vi "Microphone_input.vi"() -> ()   [LabVIEW 2013]
uses:
  <vilib>/sound2/lvsound2.llb/Sampling Mode.ctl
  <vilib>/sound2/lvsound2.llb/Sound Input Read (DBL).vi
panel:
  in  "stop":bool
  out "Waveform Graph":waveform(dbl)[](graph)
  in  "number of samples/ch":i32=100000
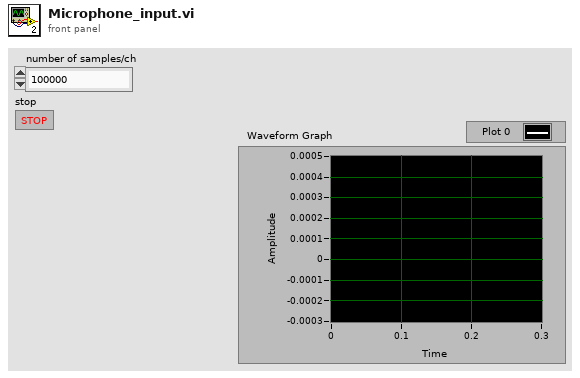
[diagram p1: front panel]
types:
  T1 = typedef "Sampling Mode.ctl" = i32
  T2 = typedef "Sound Input Task ID.ctl" = u32
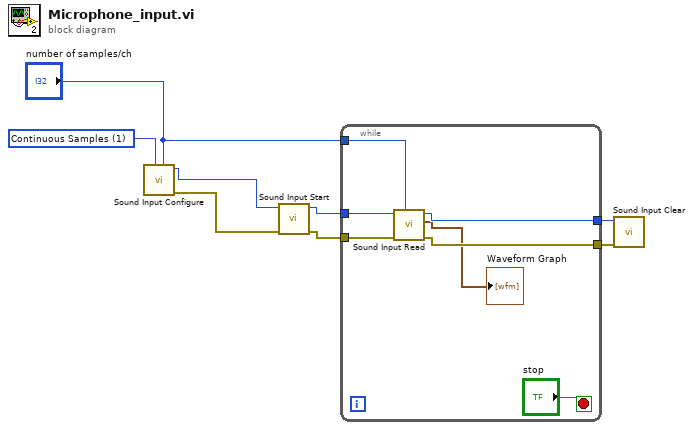
[diagram p0: block diagram]
diagram:
  w2 = T1 1 items=["Finite Samples", "Continuous Samples"] ("sample mode")
  n1 = call <vilib>:"Sound Input Configure.vi"("number of samples/ch"="number of samples/ch", "sample mode"=w2) -> ("error out"=w3:errorcluster, "task ID"=w8:T2)  [unwired: 8 in]
  n2 = call <vilib>:"Sound Input Start.vi"("error in (no error)"=w3, "task ID"=w8) -> ("error out"=w4:errorcluster, "task ID out"=w7:T2)  [unwired: 8 in]
  n3 = while {
    tunnel: w7 -> [w15]
    tunnel: [w14] -> w6
    tunnel: [w13] -> w5
    tunnel: w4 -> [w12]
    tunnel: "number of samples/ch" -> [w11]
    stop <- "stop" stop-if-true
    n4 = call-poly <vilib>:"Sound Input Read.vi"("number of samples/ch"=w11, "error in (no error)"=w12, "task ID"=w15) -> ("error out"=w13:errorcluster, "data"=→"Waveform Graph":waveform(dbl)[], "task ID out"=w14:T2)  [unwired: 6 in]
  }
  n5 = call <vilib>:"Sound Input Clear.vi"("error in (no error)"=w5, "task ID"=w6) -> ()  [unwired: 9 in, 1 out]
